vi "SP_OEE_2_test.vi"() -> ()   [LabVIEW 2017] (continued)
                      frame #2 {
                        n614 = call "Stack_holderwise_total_bd_count_&_duration.vi"("Refnum in"=w3312, "BREAKDOWN_STK_HOLD_ID"=2, "condition"=w3302, "Form Date"=w3310, "To Date"=w3309, "error in (no error)"=w3314) -> ("Refnum out"=w3311:T2, "Count out"=w3308:string[], "appended array"=w3304:dbl[], "error out"=w3313:errorcluster)  [unwired: 6 in]
                        n615 = call "Insert_empty_element_with_zero.vi"("searched date"=w3308, "fixed date"=w3305) -> ("O/P"=w3307:string[])  [unwired: 9 in]
                        n616 = call "NUMERIC TO STRING.vi"("appended array"=w3304) -> ("Array"=w3303:string[])  [unwired: 4 in]
                        n617 = call "Insert_empty_element_with_zero.vi"("searched date"=w3303, "fixed date"=w3305) -> ("O/P"=w3306:string[])  [unwired: 9 in]
                      }
                      frame #3 {
                        n618 = disable-structure shown="Enabled" {
                          disable-tunnel: w3331 -> [w3345 w3348]
                          disable-tunnel: [w3344 w3348] -> w3330
                          disable-tunnel: w3329 -> [w3343 w3347]
                          disable-tunnel: [w3342 w3347] -> w3328
                          disable-tunnel: w3327 -> [w3341 _]
                          disable-tunnel: w3326 -> [w3340 _]
                          disable-tunnel: [w3339 _] -> w3325
                          disable-tunnel: [w3338 _] -> w3321
                          disable-tunnel: w3319 -> [w3337 _]
                          frame Disabled {
                            n619 = call "Stack_holderwise_total_bd_count_&_duration.vi"("Refnum in"=w3343, "BREAKDOWN_STK_HOLD_ID"=3, "condition"=w3337, "Form Date"=w3341, "To Date"=w3340, "error in (no error)"=w3345) -> ("Refnum out"=w3342:T2, "Count out"=w3339:string[], "appended array"=w3338:dbl[], "error out"=w3344:errorcluster)  [unwired: 6 in]
                          }
                          frame Enabled {
                          }
                        }
                        n620 = call "Insert_empty_element_with_zero.vi"("searched date"=w3325, "fixed date"=w3322) -> ("O/P"=w3324:string[])  [unwired: 9 in]
                        n621 = call "NUMERIC TO STRING.vi"("appended array"=w3321) -> ("Array"=w3320:string[])  [unwired: 4 in]
                        n622 = call "Insert_empty_element_with_zero.vi"("searched date"=w3320, "fixed date"=w3322) -> ("O/P"=w3323:string[])  [unwired: 9 in]
                      }
                      frame #4 {
                        n623 = disable-structure shown="Enabled" {
                          disable-tunnel: w3362 -> [w3378 w3381]
                          disable-tunnel: w3361 -> [w3377 w3380]
                          disable-tunnel: [w3376 w3380] -> w3360
                          disable-tunnel: [w3375 w3381] -> w3359
                          disable-tunnel: w3358 -> [w3374 _]
                          disable-tunnel: w3357 -> [w3373 _]
                          disable-tunnel: [w3372 _] -> w3356
                          disable-tunnel: [w3371 _] -> w3352
                          disable-tunnel: w3350 -> [w3370 _]
                          frame Disabled {
                            n624 = call "Stack_holderwise_total_bd_count_&_duration.vi"("Refnum in"=w3377, "BREAKDOWN_STK_HOLD_ID"=4, "condition"=w3370, "Form Date"=w3374, "To Date"=w3373, "error in (no error)"=w3378) -> ("Refnum out"=w3376:T2, "Count out"=w3372:string[], "appended array"=w3371:dbl[], "error out"=w3375:errorcluster)  [unwired: 6 in]
                          }
                          frame Enabled {
                          }
                        }
                        n625 = call "Insert_empty_element_with_zero.vi"("searched date"=w3356, "fixed date"=w3353) -> ("O/P"=w3355:string[])  [unwired: 9 in]
                        n626 = call "NUMERIC TO STRING.vi"("appended array"=w3352) -> ("Array"=w3351:string[])  [unwired: 4 in]
                        n627 = call "Insert_empty_element_with_zero.vi"("searched date"=w3351, "fixed date"=w3353) -> ("O/P"=w3354:string[])  [unwired: 9 in]
                      }
                      frame #5 {
                        n628 = disable-structure shown="Enabled" {
                          disable-tunnel: w3395 -> [w3413 w3416]
                          disable-tunnel: [w3412 w3416] -> w3394
                          disable-tunnel: w3393 -> [w3411 w3415]
                          disable-tunnel: [w3410 w3415] -> w3392
                          disable-tunnel: w3391 -> [w3409 _]
                          disable-tunnel: w3390 -> [w3408 _]
                          disable-tunnel: [w3407 _] -> w3389
                          disable-tunnel: [w3406 _] -> w3385
                          disable-tunnel: w3383 -> [w3405 _]
                          frame Disabled {
                            n629 = call "Stack_holderwise_total_bd_count_&_duration.vi"("Refnum in"=w3411, "BREAKDOWN_STK_HOLD_ID"=5, "condition"=w3405, "Form Date"=w3408, "To Date"=w3409, "error in (no error)"=w3413) -> ("Refnum out"=w3410:T2, "Count out"=w3407:string[], "appended array"=w3406:dbl[], "error out"=w3412:errorcluster)  [unwired: 6 in]
                          }
                          frame Enabled {
                          }
                        }
                        n630 = call "NUMERIC TO STRING.vi"("appended array"=w3385) -> ("Array"=w3384:string[])  [unwired: 4 in]
                        n631 = call "Insert_empty_element_with_zero.vi"("searched date"=w3389, "fixed date"=w3387) -> ("O/P"=w3388:string[])  [unwired: 9 in]
                        n632 = call "Insert_empty_element_with_zero.vi"("searched date"=w3384, "fixed date"=w3387) -> ("O/P"=w3386:string[])  [unwired: 9 in]
                      }
                      frame #6 {
                        n633 = call "String to numeric.vi"("Array"=w3427) -> ("Array 2"=w3426:dbl[])  [unwired: 4 in]
                        n634 = call "String to numeric.vi"("Array"=w3425) -> ("Array 2"=w3424:dbl[])  [unwired: 4 in]
                        n635 = call "String to numeric.vi"("Array"=w3423) -> ("Array 2"=w3422:dbl[])  [unwired: 4 in]
                        n636 = call "String to numeric.vi"("Array"=w3421) -> ("Array 2"=w3420:dbl[])  [unwired: 4 in]
                        n637 = call "String to numeric.vi"("Array"=w3419) -> ("Array 2"=w3418:dbl[])  [unwired: 4 in]
                        n638 = Decimal String To Number(string=w3432) -> (number=w3451:i32[])  [unwired: 2 in, 1 out]
                        n639 = Decimal String To Number(string=w3433) -> (number=w3452:i32[])  [unwired: 2 in, 1 out]
                        n640 = Decimal String To Number(string=w3434) -> (number=w3453:i32[])  [unwired: 2 in, 1 out]
                        n641 = Decimal String To Number(string=w3435) -> (number=w3454:i32[])  [unwired: 2 in, 1 out]
                        n642 = Decimal String To Number(string=w3436) -> (number=w3449:i32[])  [unwired: 2 in, 1 out]
                        n643 = Compound Arithmetic op=ADD(w3426, w3424, w3422, w3420, w3418) -> (w3429:dbl[])
                        n644 = Build Array(w3427) -> (w3448:string[][])
                        n645 = Build Array(w3425) -> (w3447:string[][])
                        n646 = Build Array(w3423) -> (w3446:string[][])
                        n647 = Build Array(w3421) -> (w3445:string[][])
                        n648 = Build Array(w3419) -> (w3444:string[][])
                        n649 = Number To Fractional String(number=w3429, precision (6)=i16 2) -> (F-format string=w3428:string[])  [unwired: 2 in]
                        n650 = Compound Arithmetic op=ADD(w3451, w3452, w3453, w3454, w3449) -> (w3455:i32[])
                        n651 = Transpose 2D Array(2D array=w3448) -> (transposed array=w3442:string[][])
                        n652 = Transpose 2D Array(2D array=w3447) -> (transposed array=w3441:string[][])
                        n653 = Transpose 2D Array(2D array=w3446) -> (transposed array=w3440:string[][])
                        n654 = Transpose 2D Array(2D array=w3445) -> (transposed array=w3439:string[][])
                        n655 = Transpose 2D Array(2D array=w3444) -> (transposed array=w3438:string[][])
                        n656 = Number To Decimal String(number=w3455) -> (decimal integer string=w3450:string[])  [unwired: 1 in]
                        n657 = Build Array(w3428) -> (w3431:string[][])
                        n658 = Transpose 2D Array(2D array=w3431) -> (transposed array=w3437:string[][])
                      }
                      frame #7 {
                        w3458 = string[] ["0"]
                        n659 = Insert Into Array(array=w3468, index (col)=1 ("disabled index (col)"), new element #1=w3458, new element #2=w3458, new element #3=w3460, new element #4=w3459, new element #5=w3458, new element #6=w3458, new element #7=w3458, new element #8=w3458, new element #9=w3458, new element #10=w3458, new element #11=w3461, new element #12=w3462) -> (w3464:string[][])  [unwired: 1 in]
                        n660 = call "flot graph for month n year.vi"("BD Date"=w3465, "error in (no error)"=w3467, "Count total"=w3461) -> ("error out"=w3466:errorcluster, "Run-Time Status"=w3463:cluster{"Array 2":timestamp[], dbl[]})  [unwired: 7 in]
                        n661 = local write "Run-Time Status"(w3463) -> ()
                        n662 = local write "Table"(w3464) -> ()
                      }
                    }
                  }
                  frame "1" {
                    n663 = flat-sequence {
                      tunnel: w3480 -> [w3594]
                      tunnel: w3479 -> [w3592]
                      tunnel: [w3578] -> w3570
                      tunnel: [w3593] -> w3569
                      tunnel: w3478 -> [_]
                      tunnel: [w3597] -> w3568
                      tunnel: [w3577] -> w3567
                      tunnel: [w3576] -> w3566
                      tunnel: [w3575] -> w3565
                      tunnel: w3477 -> [w3577]
                      tunnel: w3476 -> [w3576]
                      tunnel: ["Where BREAKDOWN_DATE between '%s'and '%s' and BREAKDOWN_STK_HOLD_ID ='%d' and  SHIFT_ID = '%d' "] -> w3564
                      tunnel: [w3575] -> w3563
                      tunnel: w3475 -> [w3571]
                      tunnel: [w3571] -> w3474
                      tunnel: w3570 -> [w3658]
                      tunnel: w3569 -> [w3660]
                      tunnel: w3568 -> [w3656]
                      tunnel: w3567 -> [w3655]
                      tunnel: w3566 -> [w3654]
                      tunnel: [w3657] -> w3562
                      tunnel: [w3659] -> w3561
                      tunnel: [w3656] -> w3560
                      tunnel: [w3646] -> w3559
                      tunnel: [w3652] -> w3558
                      tunnel: [w3655] -> w3557
                      tunnel: [w3654] -> w3556
                      tunnel: w3565 -> [w3651]
                      tunnel: [w3651] -> w3555
                      tunnel: w3564 -> [w3648]
                      tunnel: [w3648] -> w3554
                      tunnel: [w3647] -> w3553
                      tunnel: w3563 -> [w3647]
                      tunnel: w3474 -> [w3645]
                      tunnel: [w3644] -> w3473
                      tunnel: w3562 -> [w3690]
                      tunnel: w3561 -> [w3688]
                      tunnel: w3560 -> [w3693]
                      tunnel: w3559 -> [w3692]
                      tunnel: w3558 -> [w3691]
                      tunnel: w3557 -> [w3686]
                      tunnel: w3556 -> [w3685]
                      tunnel: [w3693] -> w3552
                      tunnel: [w3692] -> w3551
                      tunnel: [w3691] -> w3550
                      tunnel: [w3689] -> w3549
                      tunnel: [w3683] -> w3548
                      tunnel: [w3682] -> w3547
                      tunnel: [w3687] -> w3546
                      tunnel: [w3686] -> w3545
                      tunnel: [w3685] -> w3544
                      tunnel: w3555 -> [w3681]
                      tunnel: [w3681] -> w3543
                      tunnel: w3554 -> [w3678]
                      tunnel: [w3678] -> w3542
                      tunnel: [w3677] -> w3541
                      tunnel: w3553 -> [w3677]
                      tunnel: w3473 -> [w3675]
                      tunnel: w3552 -> [w3712]
                      tunnel: w3551 -> [w3711]
                      tunnel: w3550 -> [w3710]
                      tunnel: w3549 -> [w3707]
                      tunnel: w3548 -> [w3709]
                      tunnel: w3547 -> [w3708]
                      tunnel: w3546 -> [w3705]
                      tunnel: w3545 -> [w3703]
                      tunnel: w3544 -> [w3702]
                      tunnel: [w3712] -> w3540
                      tunnel: [w3711] -> w3539
                      tunnel: [w3710] -> w3538
                      tunnel: [w3709] -> w3537
                      tunnel: [w3708] -> w3536
                      tunnel: [w3706] -> w3535
                      tunnel: [w3700] -> w3534
                      tunnel: [w3699] -> w3533
                      tunnel: [w3704] -> w3532
                      tunnel: [w3703] -> w3531
                      tunnel: [w3702] -> w3530
                      tunnel: w3543 -> [w3698]
                      tunnel: [w3698] -> w3529
                      tunnel: w3542 -> [w3695]
                      tunnel: [w3695] -> w3528
                      tunnel: [w3694] -> w3527
                      tunnel: w3541 -> [w3694]
                      tunnel: w3540 -> [w3745]
                      tunnel: w3539 -> [w3744]
                      tunnel: w3538 -> [w3743]
                      tunnel: w3537 -> [w3742]
                      tunnel: w3536 -> [w3741]
                      tunnel: w3535 -> [w3738]
                      tunnel: w3534 -> [w3740]
                      tunnel: w3533 -> [w3739]
                      tunnel: w3532 -> [w3737]
                      tunnel: w3531 -> [w3734]
                      tunnel: w3530 -> [w3733]
                      tunnel: [w3745] -> w3526
                      tunnel: [w3744] -> w3525
                      tunnel: [w3743] -> w3524
                      tunnel: [w3742] -> w3523
                      tunnel: [w3741] -> w3522
                      tunnel: [w3740] -> w3521
                      tunnel: [w3739] -> w3520
                      tunnel: [w3736] -> w3519
                      tunnel: [w3735] -> w3518
                      tunnel: [w3731] -> w3517
                      tunnel: [w3730] -> w3516
                      tunnel: [w3734] -> w3515
                      tunnel: [w3733] -> w3514
                      tunnel: w3529 -> [w3729]
                      tunnel: [w3729] -> w3513
                      tunnel: w3528 -> [w3726]
                      tunnel: [w3726] -> w3512
                      tunnel: [w3725] -> w3511
                      tunnel: w3527 -> [w3725]
                      tunnel: w3526 -> [w3780]
                      tunnel: w3525 -> [w3779]
                      tunnel: w3524 -> [w3778]
                      tunnel: w3523 -> [w3777]
                      tunnel: w3522 -> [w3776]
                      tunnel: w3521 -> [w3775]
                      tunnel: w3520 -> [w3774]
                      tunnel: w3519 -> [w3769]
                      tunnel: w3518 -> [w3771]
                      tunnel: w3517 -> [w3773]
                      tunnel: w3516 -> [w3772]
                      tunnel: w3515 -> [w3766]
                      tunnel: w3514 -> [w3767]
                      tunnel: [w3780] -> w3510
                      tunnel: [w3779] -> w3509
                      tunnel: [w3778] -> w3508
                      tunnel: [w3777] -> w3507
                      tunnel: [w3776] -> w3506
                      tunnel: [w3775] -> w3505
                      tunnel: [w3774] -> w3504
                      tunnel: [w3773] -> w3503
                      tunnel: [w3772] -> w3502
                      tunnel: [w3770] -> w3501
                      tunnel: [w3768] -> w3500
                      tunnel: [w3764] -> w3499
                      tunnel: [w3762] -> w3498
                      tunnel: w3513 -> [w3763]
                      tunnel: w3512 -> [w3759]
                      tunnel: [w3758] -> w3497
                      tunnel: w3511 -> [w3758]
                      tunnel: w3510 -> [w3819]
                      tunnel: w3509 -> [w3812]
                      tunnel: w3508 -> [w3803]
                      tunnel: w3507 -> [w3811]
                      tunnel: w3506 -> [w3801]
                      tunnel: w3505 -> [w3810]
                      tunnel: w3504 -> [w3799]
                      tunnel: w3503 -> [w3809]
                      tunnel: w3502 -> [w3797]
                      tunnel: w3501 -> [w3833]
                      tunnel: w3500 -> [w3832]
                      tunnel: w3499 -> [w3808]
                      tunnel: w3498 -> [w3795]
                      tunnel: [w3833] -> w3496
                      tunnel: [w3832] -> w3495
                      tunnel: [w3826] -> w3494
                      tunnel: [w3819] -> w3493
                      tunnel: [w3818] -> w3492
                      tunnel: [w3817] -> w3491
                      tunnel: [w3816] -> w3490
                      tunnel: [w3815] -> w3489
                      tunnel: [w3814] -> w3488
                      tunnel: [w3813] -> w3487
                      tunnel: [w3812] -> w3486
                      tunnel: [w3811] -> w3485
                      tunnel: [w3810] -> w3484
                      tunnel: [w3809] -> w3483
                      tunnel: [w3808] -> w3482
                      tunnel: [w3793] -> w3481
                      tunnel: w3497 -> [w3793]
                      tunnel: [w3846] -> w3471
                      tunnel: [w3834] -> _
                      tunnel: w3496 -> [w3843]
                      tunnel: w3495 -> [w3846]
                      tunnel: w3494 -> [w3838]
                      tunnel: w3493 -> [w3844]
                      tunnel: w3492 -> [_]
                      tunnel: w3491 -> [w3837]
                      tunnel: w3490 -> [_]
                      tunnel: w3489 -> [_]
                      tunnel: w3488 -> [_]
                      tunnel: w3487 -> [w3839]
                      tunnel: w3486 -> [_]
                      tunnel: w3485 -> [w3836]
                      tunnel: w3484 -> [_]
                      tunnel: w3483 -> [_]
                      tunnel: w3482 -> [_]
                      tunnel: w3481 -> [w3842]
                      tunnel: [w3834] -> w3472
                      frame #0 {
                        w3585 = "%Y-%m-%d" ("time format string (%c)")
                        n664 = Decimal String To Number(string=w3571) -> (number=w3572:i32)  [unwired: 2 in, 1 out]
                        n665 = property on="Table" class="Tbl (strict)"("Visible"=TRUE) -> ()  [unwired: 2 in, 2 out]
                        n666 = Format Date/Time String(time format string (%c)=w3585, seconds (now)=w3577) -> (date/time string=w3586:string)  [unwired: 1 in]
                        n667 = Format Date/Time String(time format string (%c)=w3585, seconds (now)=w3576) -> (date/time string=w3584:string)  [unwired: 1 in]
                        n668 = Format Into String(format string="Where BREAKDOWN_DATE between '%s' and '%s' and  SHIFT_ID = '%d'  ", w3586, w3584, w3572) -> (resulting string=w3583:string)  [unwired: 2 in, 1 out]
                        n669 = call <vilib>:"DB Tools Select Data.vi"("condition"=w3583, "error in (no error)"=w3592, "columns"=string[] ["BREAKDOWN_DATE"], "table"="STATION_1_LOG_HISTORY", "connection reference"=w3594) -> ("error out"=w3579:errorcluster, "data"=w3582:variant[][], "connection reference out"=w3593:T2)  [unwired: 1 in]
                        n670 = property on="Table 2" class="Tbl (strict)"("Visible"=FALSE) -> ()  [unwired: 2 in, 2 out]
                        n671 = xnode "Database Variant To Data"("database variant"=w3582, "error in (no error)"=w3579, "type"=string[][] [] ("Elements Found")) -> ("data"=w3580:string[][], "error out"=w3578:errorcluster)
                        n672 = Index Array(array=w3580, index (col)=0 ("disabled index (col)")) -> (element=w3588:string[])  [unwired: 1 in]
                        n673 = call "Search_1d_array_element.vi"("Count in"=string[] [] ("Elements Found"), "BD Date"=w3588, "Elements Found in"=string[] [] ("Elements Found")) -> ("Elements Found out"=w3575:string[])  [unwired: 4 in, 2 out]
                        n674 = Build Array(w3575) -> (w3598:string[][])
                        n675 = Transpose 2D Array(2D array=w3598) -> (transposed array=w3597:string[][])
                      }
                      frame #1 {
                        n676 = disable-structure shown="Enabled" {
                          disable-tunnel: w3660 -> [w3671 w3673]
                          disable-tunnel: [w3670 w3673] -> w3659
                          disable-tunnel: w3658 -> [w3669 w3674]
                          disable-tunnel: [w3668 w3674] -> w3657
                          disable-tunnel: w3655 -> [w3666 _]
                          disable-tunnel: w3654 -> [w3665 _]
                          disable-tunnel: [w3664 _] -> w3653
                          disable-tunnel: [w3663 _] -> w3650
                          disable-tunnel: w3648 -> [w3662 _]
                          disable-tunnel: w3645 -> [w3661 w3672]
                          disable-tunnel: [_ w3672] -> w3644
                          frame Disabled {
                            n677 = call "Stack_holderwise_total_bd_count_&_duration_2.vi"("Refnum in"=w3671, "BREAKDOWN_STK_HOLD_ID"=1, "condition"=w3662, "Form Date"=w3666, "To Date"=w3665, "error in (no error)"=w3669, "Shift"=w3661) -> ("Refnum out"=w3670:T2, "Count out"=w3664:string[], "appended array"=w3663:dbl[], "error out"=w3668:errorcluster)  [unwired: 5 in]
                          }
                          frame Enabled {
                          }
                        }
                        n678 = call "NUMERIC TO STRING.vi"("appended array"=w3650) -> ("Array"=w3649:string[])  [unwired: 4 in]
                        n679 = call "Insert_empty_element_with_zero.vi"("searched date"=w3653, "fixed date"=w3651) -> ("O/P"=w3646:string[])  [unwired: 9 in]
                        n680 = call "Insert_empty_element_with_zero.vi"("searched date"=w3649, "fixed date"=w3651) -> ("O/P"=w3652:string[])  [unwired: 9 in]
                      }
                      frame #2 {
                        n681 = call "Stack_holderwise_total_bd_count_&_duration_2.vi"("Refnum in"=w3688, "BREAKDOWN_STK_HOLD_ID"=2, "condition"=w3678, "Form Date"=w3686, "To Date"=w3685, "error in (no error)"=w3690, "Shift"=w3675) -> ("Refnum out"=w3687:T2, "Count out"=w3684:string[], "appended array"=w3680:dbl[], "error out"=w3689:errorcluster)  [unwired: 5 in]
                        n682 = call "Insert_empty_element_with_zero.vi"("searched date"=w3684, "fixed date"=w3681) -> ("O/P"=w3683:string[])  [unwired: 9 in]
                        n683 = call "NUMERIC TO STRING.vi"("appended array"=w3680) -> ("Array"=w3679:string[])  [unwired: 4 in]
                        n684 = call "Insert_empty_element_with_zero.vi"("searched date"=w3679, "fixed date"=w3681) -> ("O/P"=w3682:string[])  [unwired: 9 in]
                      }
                      frame #3 {
                        n685 = disable-structure shown="Enabled" {
                          disable-tunnel: w3707 -> [w3721 w3724]
                          disable-tunnel: [w3720 w3724] -> w3706
                          disable-tunnel: w3705 -> [w3719 w3723]
                          disable-tunnel: [w3718 w3723] -> w3704
                          disable-tunnel: w3703 -> [w3717 _]
                          disable-tunnel: w3702 -> [w3716 _]
                          disable-tunnel: [w3715 _] -> w3701
                          disable-tunnel: [w3714 _] -> w3697
                          disable-tunnel: w3695 -> [w3713 _]
                          frame Disabled {
                            n686 = call "Stack_holderwise_total_bd_count_&_duration.vi"("Refnum in"=w3719, "BREAKDOWN_STK_HOLD_ID"=3, "condition"=w3713, "Form Date"=w3717, "To Date"=w3716, "error in (no error)"=w3721) -> ("Refnum out"=w3718:T2, "Count out"=w3715:string[], "appended array"=w3714:dbl[], "error out"=w3720:errorcluster)  [unwired: 6 in]
                          }
                          frame Enabled {
                          }
                        }
                        n687 = call "Insert_empty_element_with_zero.vi"("searched date"=w3701, "fixed date"=w3698) -> ("O/P"=w3700:string[])  [unwired: 9 in]
                        n688 = call "NUMERIC TO STRING.vi"("appended array"=w3697) -> ("Array"=w3696:string[])  [unwired: 4 in]
                        n689 = call "Insert_empty_element_with_zero.vi"("searched date"=w3696, "fixed date"=w3698) -> ("O/P"=w3699:string[])  [unwired: 9 in]
                      }
                      frame #4 {
                        n690 = disable-structure shown="Enabled" {
                          disable-tunnel: w3738 -> [w3754 w3757]
                          disable-tunnel: w3737 -> [w3753 w3756]
                          disable-tunnel: [w3752 w3756] -> w3736
                          disable-tunnel: [w3751 w3757] -> w3735
                          disable-tunnel: w3734 -> [w3750 _]
                          disable-tunnel: w3733 -> [w3749 _]
                          disable-tunnel: [w3748 _] -> w3732
                          disable-tunnel: [w3747 _] -> w3728
                          disable-tunnel: w3726 -> [w3746 _]
                          frame Disabled {
                            n691 = call "Stack_holderwise_total_bd_count_&_duration.vi"("Refnum in"=w3753, "BREAKDOWN_STK_HOLD_ID"=4, "condition"=w3746, "Form Date"=w3750, "To Date"=w3749, "error in (no error)"=w3754) -> ("Refnum out"=w3752:T2, "Count out"=w3748:string[], "appended array"=w3747:dbl[], "error out"=w3751:errorcluster)  [unwired: 6 in]
                          }
                          frame Enabled {
                          }
                        }
                        n692 = call "Insert_empty_element_with_zero.vi"("searched date"=w3732, "fixed date"=w3729) -> ("O/P"=w3731:string[])  [unwired: 9 in]
                        n693 = call "NUMERIC TO STRING.vi"("appended array"=w3728) -> ("Array"=w3727:string[])  [unwired: 4 in]
                        n694 = call "Insert_empty_element_with_zero.vi"("searched date"=w3727, "fixed date"=w3729) -> ("O/P"=w3730:string[])  [unwired: 9 in]
                      }
                      frame #5 {
                        n695 = disable-structure shown="Enabled" {
                          disable-tunnel: w3771 -> [w3789 w3792]
                          disable-tunnel: [w3788 w3792] -> w3770
                          disable-tunnel: w3769 -> [w3787 w3791]
                          disable-tunnel: [w3786 w3791] -> w3768
                          disable-tunnel: w3767 -> [w3785 _]
                          disable-tunnel: w3766 -> [w3784 _]
                          disable-tunnel: [w3783 _] -> w3765
                          disable-tunnel: [w3782 _] -> w3761
                          disable-tunnel: w3759 -> [w3781 _]
                          frame Disabled {
                            n696 = call "Stack_holderwise_total_bd_count_&_duration.vi"("Refnum in"=w3787, "BREAKDOWN_STK_HOLD_ID"=5, "condition"=w3781, "Form Date"=w3784, "To Date"=w3785, "error in (no error)"=w3789) -> ("Refnum out"=w3786:T2, "Count out"=w3783:string[], "appended array"=w3782:dbl[], "error out"=w3788:errorcluster)  [unwired: 6 in]
                          }
                          frame Enabled {
                          }
                        }
                        n697 = call "NUMERIC TO STRING.vi"("appended array"=w3761) -> ("Array"=w3760:string[])  [unwired: 4 in]
                        n698 = call "Insert_empty_element_with_zero.vi"("searched date"=w3765, "fixed date"=w3763) -> ("O/P"=w3764:string[])  [unwired: 9 in]
                        n699 = call "Insert_empty_element_with_zero.vi"("searched date"=w3760, "fixed date"=w3763) -> ("O/P"=w3762:string[])  [unwired: 9 in]
                      }
                      frame #6 {
                        n700 = call "String to numeric.vi"("Array"=w3803) -> ("Array 2"=w3802:dbl[])  [unwired: 4 in]
                        n701 = call "String to numeric.vi"("Array"=w3801) -> ("Array 2"=w3800:dbl[])  [unwired: 4 in]
                        n702 = call "String to numeric.vi"("Array"=w3799) -> ("Array 2"=w3798:dbl[])  [unwired: 4 in]
                        n703 = call "String to numeric.vi"("Array"=w3797) -> ("Array 2"=w3796:dbl[])  [unwired: 4 in]
                        n704 = call "String to numeric.vi"("Array"=w3795) -> ("Array 2"=w3794:dbl[])  [unwired: 4 in]
                        n705 = Decimal String To Number(string=w3808) -> (number=w3827:i32[])  [unwired: 2 in, 1 out]
                        n706 = Decimal String To Number(string=w3809) -> (number=w3828:i32[])  [unwired: 2 in, 1 out]
                        n707 = Decimal String To Number(string=w3810) -> (number=w3829:i32[])  [unwired: 2 in, 1 out]
                        n708 = Decimal String To Number(string=w3811) -> (number=w3830:i32[])  [unwired: 2 in, 1 out]
                        n709 = Decimal String To Number(string=w3812) -> (number=w3825:i32[])  [unwired: 2 in, 1 out]
                        n710 = Compound Arithmetic op=ADD(w3802, w3800, w3798, w3796, w3794) -> (w3805:dbl[])
                        n711 = Build Array(w3803) -> (w3824:string[][])
                        n712 = Build Array(w3801) -> (w3823:string[][])
                        n713 = Build Array(w3799) -> (w3822:string[][])
                        n714 = Build Array(w3797) -> (w3821:string[][])
                        n715 = Build Array(w3795) -> (w3820:string[][])
                        n716 = Number To Fractional String(number=w3805, precision (6)=i16 2) -> (F-format string=w3804:string[])  [unwired: 2 in]
                        n717 = Compound Arithmetic op=ADD(w3827, w3828, w3829, w3830, w3825) -> (w3831:i32[])
                        n718 = Transpose 2D Array(2D array=w3824) -> (transposed array=w3818:string[][])
                        n719 = Transpose 2D Array(2D array=w3823) -> (transposed array=w3817:string[][])
                        n720 = Transpose 2D Array(2D array=w3822) -> (transposed array=w3816:string[][])
                        n721 = Transpose 2D Array(2D array=w3821) -> (transposed array=w3815:string[][])
                        n722 = Transpose 2D Array(2D array=w3820) -> (transposed array=w3814:string[][])
                        n723 = Number To Decimal String(number=w3831) -> (decimal integer string=w3826:string[])  [unwired: 1 in]
                        n724 = Build Array(w3804) -> (w3807:string[][])
                        n725 = Transpose 2D Array(2D array=w3807) -> (transposed array=w3813:string[][])
                      }
                      frame #7 {
                        w3835 = string[] [""]
                        n726 = Insert Into Array(array=w3844, index (col)=1 ("disabled index (col)"), new element #1=w3835, new element #2=w3835, new element #3=w3836, new element #4=w3837, new element #5=w3835, new element #6=w3835, new element #7=w3835, new element #8=w3835, new element #9=w3835, new element #10=w3835, new element #11=w3838, new element #12=w3839) -> (w3841:string[][])  [unwired: 1 in]
                        n727 = call "flot graph for month n year.vi"("BD Date"=w3842, "error in (no error)"=w3843, "Count total"=w3838) -> ("error out"=w3834:errorcluster, "Run-Time Status"=w3840:cluster{"Array 2":timestamp[], dbl[]})  [unwired: 7 in]
                        n728 = local write "Run-Time Status"(w3840) -> ()
                        n729 = local write "Table"(w3841) -> ()
                      }
                    }
                  }
                  frame "2" {
                    n730 = flat-sequence {
                      tunnel: w3856 -> [w3970]
                      tunnel: w3855 -> [w3968]
                      tunnel: [w3954] -> w3946
                      tunnel: [w3969] -> w3945
                      tunnel: w3854 -> [_]
                      tunnel: [w3973] -> w3944
                      tunnel: [w3953] -> w3943
                      tunnel: [w3952] -> w3942
                      tunnel: [w3951] -> w3941
                      tunnel: w3853 -> [w3953]
                      tunnel: w3852 -> [w3952]
                      tunnel: ["Where BREAKDOWN_DATE between '%s'and '%s' and BREAKDOWN_STK_HOLD_ID ='%d' and  SHIFT_ID = '%d' "] -> w3940
                      tunnel: [w3951] -> w3939
                      tunnel: w3851 -> [w3947]
                      tunnel: [w3947] -> w3850
                      tunnel: w3946 -> [w4034]
                      tunnel: w3945 -> [w4036]
                      tunnel: w3944 -> [w4032]
                      tunnel: w3943 -> [w4031]
                      tunnel: w3942 -> [w4030]
                      tunnel: [w4033] -> w3938
                      tunnel: [w4035] -> w3937
                      tunnel: [w4032] -> w3936
                      tunnel: [w4022] -> w3935
                      tunnel: [w4028] -> w3934
                      tunnel: [w4031] -> w3933
                      tunnel: [w4030] -> w3932
                      tunnel: w3941 -> [w4027]
                      tunnel: [w4027] -> w3931
                      tunnel: w3940 -> [w4024]
                      tunnel: [w4024] -> w3930
                      tunnel: [w4023] -> w3929
                      tunnel: w3939 -> [w4023]
                      tunnel: w3850 -> [w4021]
                      tunnel: [w4020] -> w3849
                      tunnel: w3938 -> [w4066]
                      tunnel: w3937 -> [w4064]
                      tunnel: w3936 -> [w4069]
                      tunnel: w3935 -> [w4068]
                      tunnel: w3934 -> [w4067]
                      tunnel: w3933 -> [w4062]
                      tunnel: w3932 -> [w4061]
                      tunnel: [w4069] -> w3928
                      tunnel: [w4068] -> w3927
                      tunnel: [w4067] -> w3926
                      tunnel: [w4065] -> w3925
                      tunnel: [w4059] -> w3924
                      tunnel: [w4058] -> w3923
                      tunnel: [w4063] -> w3922
                      tunnel: [w4062] -> w3921
                      tunnel: [w4061] -> w3920
                      tunnel: w3931 -> [w4057]
                      tunnel: [w4057] -> w3919
                      tunnel: w3930 -> [w4054]
                      tunnel: [w4054] -> w3918
                      tunnel: [w4053] -> w3917
                      tunnel: w3929 -> [w4053]
                      tunnel: w3849 -> [w4051]
                      tunnel: w3928 -> [w4088]
                      tunnel: w3927 -> [w4087]
                      tunnel: w3926 -> [w4086]
                      tunnel: w3925 -> [w4083]
                      tunnel: w3924 -> [w4085]
                      tunnel: w3923 -> [w4084]
                      tunnel: w3922 -> [w4081]
                      tunnel: w3921 -> [w4079]
                      tunnel: w3920 -> [w4078]
                      tunnel: [w4088] -> w3916
                      tunnel: [w4087] -> w3915
                      tunnel: [w4086] -> w3914
                      tunnel: [w4085] -> w3913
                      tunnel: [w4084] -> w3912
                      tunnel: [w4082] -> w3911
                      tunnel: [w4076] -> w3910
                      tunnel: [w4075] -> w3909
                      tunnel: [w4080] -> w3908
                      tunnel: [w4079] -> w3907
                      tunnel: [w4078] -> w3906
                      tunnel: w3919 -> [w4074]
                      tunnel: [w4074] -> w3905
                      tunnel: w3918 -> [w4071]
                      tunnel: [w4071] -> w3904
                      tunnel: [w4070] -> w3903
                      tunnel: w3917 -> [w4070]
                      tunnel: w3916 -> [w4121]
                      tunnel: w3915 -> [w4120]
                      tunnel: w3914 -> [w4119]
                      tunnel: w3913 -> [w4118]
                      tunnel: w3912 -> [w4117]
                      tunnel: w3911 -> [w4114]
                      tunnel: w3910 -> [w4116]
                      tunnel: w3909 -> [w4115]
                      tunnel: w3908 -> [w4113]
                      tunnel: w3907 -> [w4110]
                      tunnel: w3906 -> [w4109]
                      tunnel: [w4121] -> w3902
                      tunnel: [w4120] -> w3901
                      tunnel: [w4119] -> w3900
                      tunnel: [w4118] -> w3899
                      tunnel: [w4117] -> w3898
                      tunnel: [w4116] -> w3897
                      tunnel: [w4115] -> w3896
                      tunnel: [w4112] -> w3895
                      tunnel: [w4111] -> w3894
                      tunnel: [w4107] -> w3893
                      tunnel: [w4106] -> w3892
                      tunnel: [w4110] -> w3891
                      tunnel: [w4109] -> w3890
                      tunnel: w3905 -> [w4105]
                      tunnel: [w4105] -> w3889
                      tunnel: w3904 -> [w4102]
                      tunnel: [w4102] -> w3888
                      tunnel: [w4101] -> w3887
                      tunnel: w3903 -> [w4101]
                      tunnel: w3902 -> [w4156]
                      tunnel: w3901 -> [w4155]
                      tunnel: w3900 -> [w4154]
                      tunnel: w3899 -> [w4153]
                      tunnel: w3898 -> [w4152]
                      tunnel: w3897 -> [w4151]
                      tunnel: w3896 -> [w4150]
                      tunnel: w3895 -> [w4145]
                      tunnel: w3894 -> [w4147]
                      tunnel: w3893 -> [w4149]
                      tunnel: w3892 -> [w4148]
                      tunnel: w3891 -> [w4142]
                      tunnel: w3890 -> [w4143]
                      tunnel: [w4156] -> w3886
                      tunnel: [w4155] -> w3885
                      tunnel: [w4154] -> w3884
                      tunnel: [w4153] -> w3883
                      tunnel: [w4152] -> w3882
                      tunnel: [w4151] -> w3881
                      tunnel: [w4150] -> w3880
                      tunnel: [w4149] -> w3879
                      tunnel: [w4148] -> w3878
                      tunnel: [w4146] -> w3877
                      tunnel: [w4144] -> w3876
                      tunnel: [w4140] -> w3875
                      tunnel: [w4138] -> w3874
                      tunnel: w3889 -> [w4139]
                      tunnel: w3888 -> [w4135]
                      tunnel: [w4134] -> w3873
                      tunnel: w3887 -> [w4134]
                      tunnel: w3886 -> [w4195]
                      tunnel: w3885 -> [w4188]
                      tunnel: w3884 -> [w4179]
                      tunnel: w3883 -> [w4187]
                      tunnel: w3882 -> [w4177]
                      tunnel: w3881 -> [w4186]
                      tunnel: w3880 -> [w4175]
                      tunnel: w3879 -> [w4185]
                      tunnel: w3878 -> [w4173]
                      tunnel: w3877 -> [w4209]
                      tunnel: w3876 -> [w4208]
                      tunnel: w3875 -> [w4184]
                      tunnel: w3874 -> [w4171]
                      tunnel: [w4209] -> w3872
                      tunnel: [w4208] -> w3871
                      tunnel: [w4202] -> w3870
                      tunnel: [w4195] -> w3869
                      tunnel: [w4194] -> w3868
                      tunnel: [w4193] -> w3867
                      tunnel: [w4192] -> w3866
                      tunnel: [w4191] -> w3865
                      tunnel: [w4190] -> w3864
                      tunnel: [w4189] -> w3863
                      tunnel: [w4188] -> w3862
                      tunnel: [w4187] -> w3861
                      tunnel: [w4186] -> w3860
                      tunnel: [w4185] -> w3859
                      tunnel: [w4184] -> w3858
                      tunnel: [w4169] -> w3857
                      tunnel: w3873 -> [w4169]
                      tunnel: [w4222] -> w3847
                      tunnel: [w4218] -> w3848
                      tunnel: w3872 -> [w4219]
                      tunnel: w3871 -> [w4222]
                      tunnel: w3870 -> [w4213]
                      tunnel: w3869 -> [w4220]
                      tunnel: w3868 -> [_]
                      tunnel: w3867 -> [w4212]
                      tunnel: w3866 -> [_]
                      tunnel: w3865 -> [_]
                      tunnel: w3864 -> [_]
                      tunnel: w3863 -> [w4214]
                      tunnel: w3862 -> [_]
                      tunnel: w3861 -> [w4211]
                      tunnel: w3860 -> [_]
                      tunnel: w3859 -> [_]
                      tunnel: w3858 -> [_]
                      tunnel: w3857 -> [w4217]
                      frame #0 {
                        w3961 = "%Y-%m-%d" ("time format string (%c)")
                        n731 = Decimal String To Number(string=w3947) -> (number=w3948:i32)  [unwired: 2 in, 1 out]
                        n732 = property on="Table" class="Tbl (strict)"("Visible"=TRUE) -> ()  [unwired: 2 in, 2 out]
                        n733 = Format Date/Time String(time format string (%c)=w3961, seconds (now)=w3953) -> (date/time string=w3962:string)  [unwired: 1 in]
                        n734 = Format Date/Time String(time format string (%c)=w3961, seconds (now)=w3952) -> (date/time string=w3960:string)  [unwired: 1 in]
                        n735 = Format Into String(format string="Where BREAKDOWN_DATE between '%s' and '%s' and  SHIFT_ID = '%d'  ", w3962, w3960, w3948) -> (resulting string=w3959:string)  [unwired: 2 in, 1 out]
                        n736 = call <vilib>:"DB Tools Select Data.vi"("condition"=w3959, "error in (no error)"=w3968, "columns"=string[] ["BREAKDOWN_DATE"], "table"="STATION_1_LOG_HISTORY", "connection reference"=w3970) -> ("error out"=w3955:errorcluster, "data"=w3958:variant[][], "connection reference out"=w3969:T2)  [unwired: 1 in]
                        n737 = property on="Table 2" class="Tbl (strict)"("Visible"=FALSE) -> ()  [unwired: 2 in, 2 out]
                        n738 = xnode "Database Variant To Data"("database variant"=w3958, "error in (no error)"=w3955, "type"=string[][] [] ("Elements Found")) -> ("data"=w3956:string[][], "error out"=w3954:errorcluster)
                        n739 = Index Array(array=w3956, index (col)=0 ("disabled index (col)")) -> (element=w3964:string[])  [unwired: 1 in]
                        n740 = call "Search_1d_array_element.vi"("Count in"=string[] [] ("Elements Found"), "BD Date"=w3964, "Elements Found in"=string[] [] ("Elements Found")) -> ("Elements Found out"=w3951:string[])  [unwired: 4 in, 2 out]
                        n741 = Build Array(w3951) -> (w3974:string[][])
                        n742 = Transpose 2D Array(2D array=w3974) -> (transposed array=w3973:string[][])
                      }
                      frame #1 {
                        n743 = disable-structure shown="Enabled" {
                          disable-tunnel: w4036 -> [w4047 w4049]
                          disable-tunnel: [w4046 w4049] -> w4035
                          disable-tunnel: w4034 -> [w4045 w4050]
                          disable-tunnel: [w4044 w4050] -> w4033
                          disable-tunnel: w4031 -> [w4042 _]
                          disable-tunnel: w4030 -> [w4041 _]
                          disable-tunnel: [w4040 _] -> w4029
                          disable-tunnel: [w4039 _] -> w4026
                          disable-tunnel: w4024 -> [w4038 _]
                          disable-tunnel: w4021 -> [w4037 w4048]
                          disable-tunnel: [_ w4048] -> w4020
                          frame Disabled {
                            n744 = call "Stack_holderwise_total_bd_count_&_duration_2.vi"("Refnum in"=w4047, "BREAKDOWN_STK_HOLD_ID"=1, "condition"=w4038, "Form Date"=w4042, "To Date"=w4041, "error in (no error)"=w4045, "Shift"=w4037) -> ("Refnum out"=w4046:T2, "Count out"=w4040:string[], "appended array"=w4039:dbl[], "error out"=w4044:errorcluster)  [unwired: 5 in]
                          }
                          frame Enabled {
                          }
                        }
                        n745 = call "NUMERIC TO STRING.vi"("appended array"=w4026) -> ("Array"=w4025:string[])  [unwired: 4 in]
                        n746 = call "Insert_empty_element_with_zero.vi"("searched date"=w4029, "fixed date"=w4027) -> ("O/P"=w4022:string[])  [unwired: 9 in]
                        n747 = call "Insert_empty_element_with_zero.vi"("searched date"=w4025, "fixed date"=w4027) -> ("O/P"=w4028:string[])  [unwired: 9 in]
                      }
                      frame #2 {
                        n748 = call "Stack_holderwise_total_bd_count_&_duration_2.vi"("Refnum in"=w4064, "BREAKDOWN_STK_HOLD_ID"=2, "condition"=w4054, "Form Date"=w4062, "To Date"=w4061, "error in (no error)"=w4066, "Shift"=w4051) -> ("Refnum out"=w4063:T2, "Count out"=w4060:string[], "appended array"=w4056:dbl[], "error out"=w4065:errorcluster)  [unwired: 5 in]
                        n749 = call "Insert_empty_element_with_zero.vi"("searched date"=w4060, "fixed date"=w4057) -> ("O/P"=w4059:string[])  [unwired: 9 in]
                        n750 = call "NUMERIC TO STRING.vi"("appended array"=w4056) -> ("Array"=w4055:string[])  [unwired: 4 in]
                        n751 = call "Insert_empty_element_with_zero.vi"("searched date"=w4055, "fixed date"=w4057) -> ("O/P"=w4058:string[])  [unwired: 9 in]
                      }
                      frame #3 {
                        n752 = disable-structure shown="Enabled" {
                          disable-tunnel: w4083 -> [w4097 w4100]
                          disable-tunnel: [w4096 w4100] -> w4082
                          disable-tunnel: w4081 -> [w4095 w4099]
                          disable-tunnel: [w4094 w4099] -> w4080
                          disable-tunnel: w4079 -> [w4093 _]
                          disable-tunnel: w4078 -> [w4092 _]
                          disable-tunnel: [w4091 _] -> w4077
                          disable-tunnel: [w4090 _] -> w4073
                          disable-tunnel: w4071 -> [w4089 _]
                          frame Disabled {
                            n753 = call "Stack_holderwise_total_bd_count_&_duration.vi"("Refnum in"=w4095, "BREAKDOWN_STK_HOLD_ID"=3, "condition"=w4089, "Form Date"=w4093, "To Date"=w4092, "error in (no error)"=w4097) -> ("Refnum out"=w4094:T2, "Count out"=w4091:string[], "appended array"=w4090:dbl[], "error out"=w4096:errorcluster)  [unwired: 6 in]
                          }
                          frame Enabled {
                          }
                        }
                        n754 = call "Insert_empty_element_with_zero.vi"("searched date"=w4077, "fixed date"=w4074) -> ("O/P"=w4076:string[])  [unwired: 9 in]
                        n755 = call "NUMERIC TO STRING.vi"("appended array"=w4073) -> ("Array"=w4072:string[])  [unwired: 4 in]
                        n756 = call "Insert_empty_element_with_zero.vi"("searched date"=w4072, "fixed date"=w4074) -> ("O/P"=w4075:string[])  [unwired: 9 in]
                      }
                      frame #4 {
                        n757 = disable-structure shown="Enabled" {
                          disable-tunnel: w4114 -> [w4130 w4133]
                          disable-tunnel: w4113 -> [w4129 w4132]
                          disable-tunnel: [w4128 w4132] -> w4112
                          disable-tunnel: [w4127 w4133] -> w4111
                          disable-tunnel: w4110 -> [w4126 _]
                          disable-tunnel: w4109 -> [w4125 _]
                          disable-tunnel: [w4124 _] -> w4108
                          disable-tunnel: [w4123 _] -> w4104
                          disable-tunnel: w4102 -> [w4122 _]
                          frame Disabled {
                            n758 = call "Stack_holderwise_total_bd_count_&_duration.vi"("Refnum in"=w4129, "BREAKDOWN_STK_HOLD_ID"=4, "condition"=w4122, "Form Date"=w4126, "To Date"=w4125, "error in (no error)"=w4130) -> ("Refnum out"=w4128:T2, "Count out"=w4124:string[], "appended array"=w4123:dbl[], "error out"=w4127:errorcluster)  [unwired: 6 in]
                          }
                          frame Enabled {
                          }
                        }
                        n759 = call "Insert_empty_element_with_zero.vi"("searched date"=w4108, "fixed date"=w4105) -> ("O/P"=w4107:string[])  [unwired: 9 in]
                        n760 = call "NUMERIC TO STRING.vi"("appended array"=w4104) -> ("Array"=w4103:string[])  [unwired: 4 in]
                        n761 = call "Insert_empty_element_with_zero.vi"("searched date"=w4103, "fixed date"=w4105) -> ("O/P"=w4106:string[])  [unwired: 9 in]
                      }
                      frame #5 {
                        n762 = disable-structure shown="Enabled" {
                          disable-tunnel: w4147 -> [w4165 w4168]
                          disable-tunnel: [w4164 w4168] -> w4146
                          disable-tunnel: w4145 -> [w4163 w4167]
                          disable-tunnel: [w4162 w4167] -> w4144
                          disable-tunnel: w4143 -> [w4161 _]
                          disable-tunnel: w4142 -> [w4160 _]
                          disable-tunnel: [w4159 _] -> w4141
                          disable-tunnel: [w4158 _] -> w4137
                          disable-tunnel: w4135 -> [w4157 _]
                          frame Disabled {
                            n763 = call "Stack_holderwise_total_bd_count_&_duration.vi"("Refnum in"=w4163, "BREAKDOWN_STK_HOLD_ID"=5, "condition"=w4157, "Form Date"=w4160, "To Date"=w4161, "error in (no error)"=w4165) -> ("Refnum out"=w4162:T2, "Count out"=w4159:string[], "appended array"=w4158:dbl[], "error out"=w4164:errorcluster)  [unwired: 6 in]
                          }
                          frame Enabled {
                          }
                        }
                        n764 = call "NUMERIC TO STRING.vi"("appended array"=w4137) -> ("Array"=w4136:string[])  [unwired: 4 in]
                        n765 = call "Insert_empty_element_with_zero.vi"("searched date"=w4141, "fixed date"=w4139) -> ("O/P"=w4140:string[])  [unwired: 9 in]
                        n766 = call "Insert_empty_element_with_zero.vi"("searched date"=w4136, "fixed date"=w4139) -> ("O/P"=w4138:string[])  [unwired: 9 in]
                      }
                      frame #6 {
                        n767 = call "String to numeric.vi"("Array"=w4179) -> ("Array 2"=w4178:dbl[])  [unwired: 4 in]
                        n768 = call "String to numeric.vi"("Array"=w4177) -> ("Array 2"=w4176:dbl[])  [unwired: 4 in]
                        n769 = call "String to numeric.vi"("Array"=w4175) -> ("Array 2"=w4174:dbl[])  [unwired: 4 in]
                        n770 = call "String to numeric.vi"("Array"=w4173) -> ("Array 2"=w4172:dbl[])  [unwired: 4 in]
                        n771 = call "String to numeric.vi"("Array"=w4171) -> ("Array 2"=w4170:dbl[])  [unwired: 4 in]
                        n772 = Decimal String To Number(string=w4184) -> (number=w4203:i32[])  [unwired: 2 in, 1 out]
                        n773 = Decimal String To Number(string=w4185) -> (number=w4204:i32[])  [unwired: 2 in, 1 out]
                        n774 = Decimal String To Number(string=w4186) -> (number=w4205:i32[])  [unwired: 2 in, 1 out]
                        n775 = Decimal String To Number(string=w4187) -> (number=w4206:i32[])  [unwired: 2 in, 1 out]
                        n776 = Decimal String To Number(string=w4188) -> (number=w4201:i32[])  [unwired: 2 in, 1 out]
                        n777 = Compound Arithmetic op=ADD(w4178, w4176, w4174, w4172, w4170) -> (w4181:dbl[])
                        n778 = Build Array(w4179) -> (w4200:string[][])
                        n779 = Build Array(w4177) -> (w4199:string[][])
                        n780 = Build Array(w4175) -> (w4198:string[][])
                        n781 = Build Array(w4173) -> (w4197:string[][])
                        n782 = Build Array(w4171) -> (w4196:string[][])
                        n783 = Number To Fractional String(number=w4181, precision (6)=i16 2) -> (F-format string=w4180:string[])  [unwired: 2 in]
                        n784 = Compound Arithmetic op=ADD(w4203, w4204, w4205, w4206, w4201) -> (w4207:i32[])
                        n785 = Transpose 2D Array(2D array=w4200) -> (transposed array=w4194:string[][])
                        n786 = Transpose 2D Array(2D array=w4199) -> (transposed array=w4193:string[][])
                        n787 = Transpose 2D Array(2D array=w4198) -> (transposed array=w4192:string[][])
                        n788 = Transpose 2D Array(2D array=w4197) -> (transposed array=w4191:string[][])
                        n789 = Transpose 2D Array(2D array=w4196) -> (transposed array=w4190:string[][])
                        n790 = Number To Decimal String(number=w4207) -> (decimal integer string=w4202:string[])  [unwired: 1 in]
                        n791 = Build Array(w4180) -> (w4183:string[][])
                        n792 = Transpose 2D Array(2D array=w4183) -> (transposed array=w4189:string[][])
                      }
                      frame #7 {
                        w4210 = string[] [""]
                        n793 = Insert Into Array(array=w4220, index (col)=1 ("disabled index (col)"), new element #1=w4210, new element #2=w4210, new element #3=w4211, new element #4=w4212, new element #5=w4210, new element #6=w4210, new element #7=w4210, new element #8=w4210, new element #9=w4210, new element #10=w4210, new element #11=w4213, new element #12=w4214) -> (w4216:string[][])  [unwired: 1 in]
                        n794 = call "flot graph for month n year.vi"("BD Date"=w4217, "error in (no error)"=w4219, "Count total"=w4213) -> ("error out"=w4218:errorcluster, "Run-Time Status"=w4215:cluster{"Array 2":timestamp[], dbl[]})  [unwired: 7 in]
                        n795 = local write "Run-Time Status"(w4215) -> ()
                        n796 = local write "Table"(w4216) -> ()
                      }
                    }
                  }
                  frame "3" {
                    n797 = flat-sequence {
                      tunnel: w4232 -> [w4346]
                      tunnel: w4231 -> [w4344]
                      tunnel: [w4330] -> w4322
                      tunnel: [w4345] -> w4321
                      tunnel: w4230 -> [_]
                      tunnel: [w4349] -> w4320
                      tunnel: [w4329] -> w4319
                      tunnel: [w4328] -> w4318
                      tunnel: [w4327] -> w4317
                      tunnel: w4229 -> [w4329]
                      tunnel: w4228 -> [w4328]
                      tunnel: ["Where BREAKDOWN_DATE between '%s'and '%s' and BREAKDOWN_STK_HOLD_ID ='%d' and  SHIFT_ID = '%d' "] -> w4316
                      tunnel: [w4327] -> w4315
                      tunnel: w4227 -> [w4323]
                      tunnel: [w4323] -> w4226
                      tunnel: w4322 -> [w4410]
                      tunnel: w4321 -> [w4412]
                      tunnel: w4320 -> [w4408]
                      tunnel: w4319 -> [w4407]
                      tunnel: w4318 -> [w4406]
                      tunnel: [w4409] -> w4314
                      tunnel: [w4411] -> w4313
                      tunnel: [w4408] -> w4312
                      tunnel: [w4398] -> w4311
                      tunnel: [w4404] -> w4310
                      tunnel: [w4407] -> w4309
                      tunnel: [w4406] -> w4308
                      tunnel: w4317 -> [w4403]
                      tunnel: [w4403] -> w4307
                      tunnel: w4316 -> [w4400]
                      tunnel: [w4400] -> w4306
                      tunnel: [w4399] -> w4305
                      tunnel: w4315 -> [w4399]
                      tunnel: w4226 -> [w4397]
                      tunnel: [w4396] -> w4225
                      tunnel: w4314 -> [w4442]
                      tunnel: w4313 -> [w4440]
                      tunnel: w4312 -> [w4445]
                      tunnel: w4311 -> [w4444]
                      tunnel: w4310 -> [w4443]
                      tunnel: w4309 -> [w4438]
                      tunnel: w4308 -> [w4437]
                      tunnel: [w4445] -> w4304
                      tunnel: [w4444] -> w4303
                      tunnel: [w4443] -> w4302
                      tunnel: [w4441] -> w4301
                      tunnel: [w4435] -> w4300
                      tunnel: [w4434] -> w4299
                      tunnel: [w4439] -> w4298
                      tunnel: [w4438] -> w4297
                      tunnel: [w4437] -> w4296
                      tunnel: w4307 -> [w4433]
                      tunnel: [w4433] -> w4295
                      tunnel: w4306 -> [w4430]
                      tunnel: [w4430] -> w4294
                      tunnel: [w4429] -> w4293
                      tunnel: w4305 -> [w4429]
                      tunnel: w4225 -> [w4427]
                      tunnel: w4304 -> [w4464]
                      tunnel: w4303 -> [w4463]
                      tunnel: w4302 -> [w4462]
                      tunnel: w4301 -> [w4459]
                      tunnel: w4300 -> [w4461]
                      tunnel: w4299 -> [w4460]
                      tunnel: w4298 -> [w4457]
                      tunnel: w4297 -> [w4455]
                      tunnel: w4296 -> [w4454]
                      tunnel: [w4464] -> w4292
                      tunnel: [w4463] -> w4291
                      tunnel: [w4462] -> w4290
                      tunnel: [w4461] -> w4289
                      tunnel: [w4460] -> w4288
                      tunnel: [w4458] -> w4287
                      tunnel: [w4452] -> w4286
                      tunnel: [w4451] -> w4285
                      tunnel: [w4456] -> w4284
                      tunnel: [w4455] -> w4283
                      tunnel: [w4454] -> w4282
                      tunnel: w4295 -> [w4450]
                      tunnel: [w4450] -> w4281
                      tunnel: w4294 -> [w4447]
                      tunnel: [w4447] -> w4280
                      tunnel: [w4446] -> w4279
                      tunnel: w4293 -> [w4446]
                      tunnel: w4292 -> [w4497]
                      tunnel: w4291 -> [w4496]
                      tunnel: w4290 -> [w4495]
                      tunnel: w4289 -> [w4494]
                      tunnel: w4288 -> [w4493]
                      tunnel: w4287 -> [w4490]
                      tunnel: w4286 -> [w4492]
                      tunnel: w4285 -> [w4491]
                      tunnel: w4284 -> [w4489]
                      tunnel: w4283 -> [w4486]
                      tunnel: w4282 -> [w4485]
                      tunnel: [w4497] -> w4278
                      tunnel: [w4496] -> w4277
                      tunnel: [w4495] -> w4276
                      tunnel: [w4494] -> w4275
                      tunnel: [w4493] -> w4274
                      tunnel: [w4492] -> w4273
                      tunnel: [w4491] -> w4272
                      tunnel: [w4488] -> w4271
                      tunnel: [w4487] -> w4270
                      tunnel: [w4483] -> w4269
                      tunnel: [w4482] -> w4268
                      tunnel: [w4486] -> w4267
                      tunnel: [w4485] -> w4266
                      tunnel: w4281 -> [w4481]
                      tunnel: [w4481] -> w4265
                      tunnel: w4280 -> [w4478]
                      tunnel: [w4478] -> w4264
                      tunnel: [w4477] -> w4263
                      tunnel: w4279 -> [w4477]
                      tunnel: w4278 -> [w4532]
                      tunnel: w4277 -> [w4531]
                      tunnel: w4276 -> [w4530]
                      tunnel: w4275 -> [w4529]
                      tunnel: w4274 -> [w4528]
                      tunnel: w4273 -> [w4527]
                      tunnel: w4272 -> [w4526]
                      tunnel: w4271 -> [w4521]
                      tunnel: w4270 -> [w4523]
                      tunnel: w4269 -> [w4525]
                      tunnel: w4268 -> [w4524]
                      tunnel: w4267 -> [w4518]
                      tunnel: w4266 -> [w4519]
                      tunnel: [w4532] -> w4262
                      tunnel: [w4531] -> w4261
                      tunnel: [w4530] -> w4260
                      tunnel: [w4529] -> w4259
                      tunnel: [w4528] -> w4258
                      tunnel: [w4527] -> w4257
                      tunnel: [w4526] -> w4256
                      tunnel: [w4525] -> w4255
                      tunnel: [w4524] -> w4254
                      tunnel: [w4522] -> w4253
                      tunnel: [w4520] -> w4252
                      tunnel: [w4516] -> w4251
                      tunnel: [w4514] -> w4250
                      tunnel: w4265 -> [w4515]
                      tunnel: w4264 -> [w4511]
                      tunnel: [w4510] -> w4249
                      tunnel: w4263 -> [w4510]
                      tunnel: w4262 -> [w4571]
                      tunnel: w4261 -> [w4564]
                      tunnel: w4260 -> [w4555]
                      tunnel: w4259 -> [w4563]
                      tunnel: w4258 -> [w4553]
                      tunnel: w4257 -> [w4562]
                      tunnel: w4256 -> [w4551]
                      tunnel: w4255 -> [w4561]
                      tunnel: w4254 -> [w4549]
                      tunnel: w4253 -> [w4585]
                      tunnel: w4252 -> [w4584]
                      tunnel: w4251 -> [w4560]
                      tunnel: w4250 -> [w4547]
                      tunnel: [w4585] -> w4248
                      tunnel: [w4584] -> w4247
                      tunnel: [w4578] -> w4246
                      tunnel: [w4571] -> w4245
                      tunnel: [w4570] -> w4244
                      tunnel: [w4569] -> w4243
                      tunnel: [w4568] -> w4242
                      tunnel: [w4567] -> w4241
                      tunnel: [w4566] -> w4240
                      tunnel: [w4565] -> w4239
                      tunnel: [w4564] -> w4238
                      tunnel: [w4563] -> w4237
                      tunnel: [w4562] -> w4236
                      tunnel: [w4561] -> w4235
                      tunnel: [w4560] -> w4234
                      tunnel: [w4545] -> w4233
                      tunnel: w4249 -> [w4545]
                      tunnel: [w4586] -> _
                      tunnel: [w4595] -> w4223
                      tunnel: w4248 -> [w4596]
                      tunnel: w4247 -> [w4586]
                      tunnel: w4246 -> [w4590]
                      tunnel: w4245 -> [w4597]
                      tunnel: w4244 -> [_]
                      tunnel: w4243 -> [w4589]
                      tunnel: w4242 -> [_]
                      tunnel: w4241 -> [_]
                      tunnel: w4240 -> [_]
                      tunnel: w4239 -> [w4591]
                      tunnel: w4238 -> [_]
                      tunnel: w4237 -> [w4588]
                      tunnel: w4236 -> [_]
                      tunnel: w4235 -> [_]
                      tunnel: w4234 -> [_]
                      tunnel: w4233 -> [w4594]
                      tunnel: [w4586] -> w4224
                      frame #0 {
                        w4337 = "%Y-%m-%d" ("time format string (%c)")
                        n798 = Decimal String To Number(string=w4323) -> (number=w4324:i32)  [unwired: 2 in, 1 out]
                        n799 = property on="Table" class="Tbl (strict)"("Visible"=TRUE) -> ()  [unwired: 2 in, 2 out]
                        n800 = Format Date/Time String(time format string (%c)=w4337, seconds (now)=w4329) -> (date/time string=w4338:string)  [unwired: 1 in]
                        n801 = Format Date/Time String(time format string (%c)=w4337, seconds (now)=w4328) -> (date/time string=w4336:string)  [unwired: 1 in]
                        n802 = Format Into String(format string="Where BREAKDOWN_DATE between '%s' and '%s' and  SHIFT_ID = '%d'  ", w4338, w4336, w4324) -> (resulting string=w4335:string)  [unwired: 2 in, 1 out]
                        n803 = call <vilib>:"DB Tools Select Data.vi"("condition"=w4335, "error in (no error)"=w4344, "columns"=string[] ["BREAKDOWN_DATE"], "table"="STATION_1_LOG_HISTORY", "connection reference"=w4346) -> ("error out"=w4331:errorcluster, "data"=w4334:variant[][], "connection reference out"=w4345:T2)  [unwired: 1 in]
                        n804 = property on="Table 2" class="Tbl (strict)"("Visible"=FALSE) -> ()  [unwired: 2 in, 2 out]
                        n805 = xnode "Database Variant To Data"("database variant"=w4334, "error in (no error)"=w4331, "type"=string[][] [] ("Elements Found")) -> ("data"=w4332:string[][], "error out"=w4330:errorcluster)
                        n806 = Index Array(array=w4332, index (col)=0 ("disabled index (col)")) -> (element=w4340:string[])  [unwired: 1 in]
                        n807 = call "Search_1d_array_element.vi"("Count in"=string[] [] ("Elements Found"), "BD Date"=w4340, "Elements Found in"=string[] [] ("Elements Found")) -> ("Elements Found out"=w4327:string[])  [unwired: 4 in, 2 out]
                        n808 = Build Array(w4327) -> (w4350:string[][])
                        n809 = Transpose 2D Array(2D array=w4350) -> (transposed array=w4349:string[][])
                      }
                      frame #1 {
                        n810 = disable-structure shown="Enabled" {
                          disable-tunnel: w4412 -> [w4423 w4425]
                          disable-tunnel: [w4422 w4425] -> w4411
                          disable-tunnel: w4410 -> [w4421 w4426]
                          disable-tunnel: [w4420 w4426] -> w4409
                          disable-tunnel: w4407 -> [w4418 _]
                          disable-tunnel: w4406 -> [w4417 _]
                          disable-tunnel: [w4416 _] -> w4405
                          disable-tunnel: [w4415 _] -> w4402
                          disable-tunnel: w4400 -> [w4414 _]
                          disable-tunnel: w4397 -> [w4413 w4424]
                          disable-tunnel: [_ w4424] -> w4396
                          frame Disabled {
                            n811 = call "Stack_holderwise_total_bd_count_&_duration_2.vi"("Refnum in"=w4423, "BREAKDOWN_STK_HOLD_ID"=1, "condition"=w4414, "Form Date"=w4418, "To Date"=w4417, "error in (no error)"=w4421, "Shift"=w4413) -> ("Refnum out"=w4422:T2, "Count out"=w4416:string[], "appended array"=w4415:dbl[], "error out"=w4420:errorcluster)  [unwired: 5 in]
                          }
                          frame Enabled {
                          }
                        }
                        n812 = call "NUMERIC TO STRING.vi"("appended array"=w4402) -> ("Array"=w4401:string[])  [unwired: 4 in]
                        n813 = call "Insert_empty_element_with_zero.vi"("searched date"=w4405, "fixed date"=w4403) -> ("O/P"=w4398:string[])  [unwired: 9 in]
                        n814 = call "Insert_empty_element_with_zero.vi"("searched date"=w4401, "fixed date"=w4403) -> ("O/P"=w4404:string[])  [unwired: 9 in]
                      }
                      frame #2 {
                        n815 = call "Stack_holderwise_total_bd_count_&_duration_2.vi"("Refnum in"=w4440, "BREAKDOWN_STK_HOLD_ID"=2, "condition"=w4430, "Form Date"=w4438, "To Date"=w4437, "error in (no error)"=w4442, "Shift"=w4427) -> ("Refnum out"=w4439:T2, "Count out"=w4436:string[], "appended array"=w4432:dbl[], "error out"=w4441:errorcluster)  [unwired: 5 in]
                        n816 = call "Insert_empty_element_with_zero.vi"("searched date"=w4436, "fixed date"=w4433) -> ("O/P"=w4435:string[])  [unwired: 9 in]
                        n817 = call "NUMERIC TO STRING.vi"("appended array"=w4432) -> ("Array"=w4431:string[])  [unwired: 4 in]
                        n818 = call "Insert_empty_element_with_zero.vi"("searched date"=w4431, "fixed date"=w4433) -> ("O/P"=w4434:string[])  [unwired: 9 in]
                      }
                      frame #3 {
                        n819 = disable-structure shown="Enabled" {
                          disable-tunnel: w4459 -> [w4473 w4476]
                          disable-tunnel: [w4472 w4476] -> w4458
                          disable-tunnel: w4457 -> [w4471 w4475]
                          disable-tunnel: [w4470 w4475] -> w4456
                          disable-tunnel: w4455 -> [w4469 _]
                          disable-tunnel: w4454 -> [w4468 _]
                          disable-tunnel: [w4467 _] -> w4453
                          disable-tunnel: [w4466 _] -> w4449
                          disable-tunnel: w4447 -> [w4465 _]
                          frame Disabled {
                            n820 = call "Stack_holderwise_total_bd_count_&_duration.vi"("Refnum in"=w4471, "BREAKDOWN_STK_HOLD_ID"=3, "condition"=w4465, "Form Date"=w4469, "To Date"=w4468, "error in (no error)"=w4473) -> ("Refnum out"=w4470:T2, "Count out"=w4467:string[], "appended array"=w4466:dbl[], "error out"=w4472:errorcluster)  [unwired: 6 in]
                          }
                          frame Enabled {
                          }
                        }
                        n821 = call "Insert_empty_element_with_zero.vi"("searched date"=w4453, "fixed date"=w4450) -> ("O/P"=w4452:string[])  [unwired: 9 in]
                        n822 = call "NUMERIC TO STRING.vi"("appended array"=w4449) -> ("Array"=w4448:string[])  [unwired: 4 in]
                        n823 = call "Insert_empty_element_with_zero.vi"("searched date"=w4448, "fixed date"=w4450) -> ("O/P"=w4451:string[])  [unwired: 9 in]
                      }
                      frame #4 {
                        n824 = disable-structure shown="Enabled" {
                          disable-tunnel: w4490 -> [w4506 w4509]
